vi "Roller DB Update.vi"   [LabVIEW 2014]
uses:
  Robot Global Data.vi
types:
  T1 = typedef "Dashboard Control Data.ctl" = cluster{"Cam Exposure":dbl, "Go to angle":dbl, "PID gains":cluster{"proportional gain (Kc)":dbl, "integral time (Ti, min)":dbl, "derivative time (Td, min)":dbl}, "output range":cluster{"output high":dbl, "output low":dbl}, "Pressure m \nValue":dbl, "Pressure b \nValue":dbl, "Strafe Timer\nWait":dbl, "Roller Command Cluster ":T2}
  T2 = typedef "Roller Control.ctl" = cluster{"Mode":enum16{"Manual", "Idle", "Grab Tote", "Align Tote", "Load Tote", "Unload Totes"}, "Tote Inside?":bool, "Claw Piston":bool, "Manual":cluster{"Manual Claw":bool, "Right Roller":bool, "Left Roller":bool, "Left Roller Back":bool, "Right Roller Back":bool}, "Left Roller Speed":dbl, "Right Roller Speed":dbl, "Left Roller Speed Back":dbl, "Right Roller Speed Back":dbl}
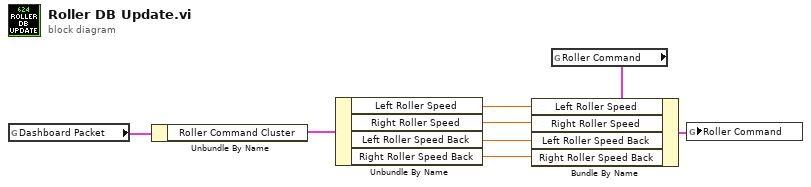
[diagram p0: block diagram]
diagram:
  n1 = global read "Robot Global Data.vi" "Dashboard Packet"() -> (w8:T1)
  n2 = Unbundle By Name(w8) -> ("Roller Command Cluster"=w7:T2)
  n3 = Unbundle By Name(w7) -> ("Left Roller Speed"=w4:dbl, "Right Roller Speed"=w3:dbl, "Left Roller Speed Back"=w2:dbl, "Right Roller Speed Back"=w1:dbl)
  n4 = global read "Robot Global Data.vi" "Roller Command"() -> (w6:T2)
  n5 = Bundle By Name(cluster=w6, "Left Roller Speed"=w4, "Right Roller Speed"=w3, "Left Roller Speed Back"=w2, "Right Roller Speed Back"=w1) -> (w5:T2)
  n6 = global write "Robot Global Data.vi" "Roller Command"(w5) -> ()
